vi "MainVI.vi"() -> ()   [LabVIEW 2020]
uses:
  System.Speech
panel:
  in  "WITHDRAW":bool
  in  "PIN ENTER":bool
  in  "Keyboard":T1
  in  "NAME ENTER":bool
  in  "RUN":bool
  in  "INSERT CARD":bool
  out "Screen":string
  # "PROJECT"
  # "VIRTUAL ATM"
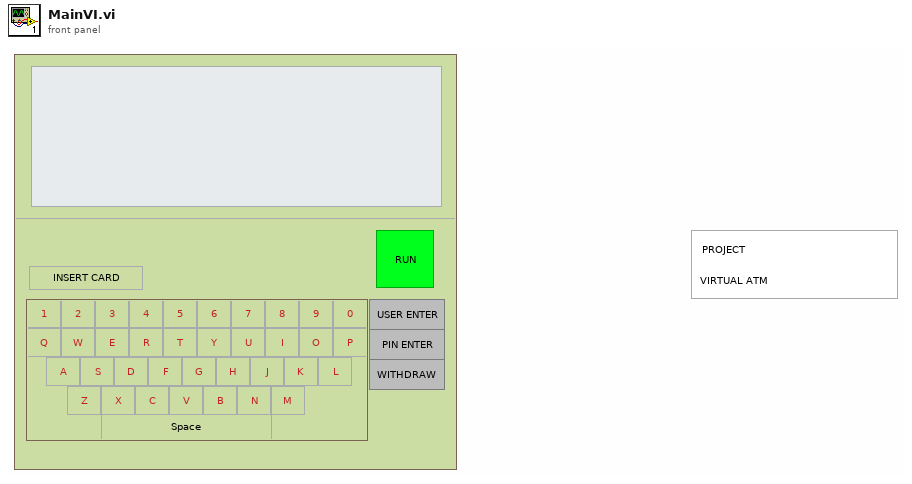
[diagram p1: front panel]
types:
  T1 = cluster{"Q":bool, "W":bool, "E":bool, "R":bool, "T":bool, "Y":bool, "U":bool, "I":bool, "O":bool, "P":bool, "A":bool, "S":bool, "D":bool, "F":bool, "G":bool, "H":bool, "J":bool, "K":bool, "L":bool, "Z":bool, "X":bool, "C":bool, "V":bool, "B":bool, "N":bool, "M":bool, "1":bool, "2":bool, "3":bool, "4":bool, "5":bool, "6":bool, "7":bool, "8":bool, "9":bool, "0":bool, bool}
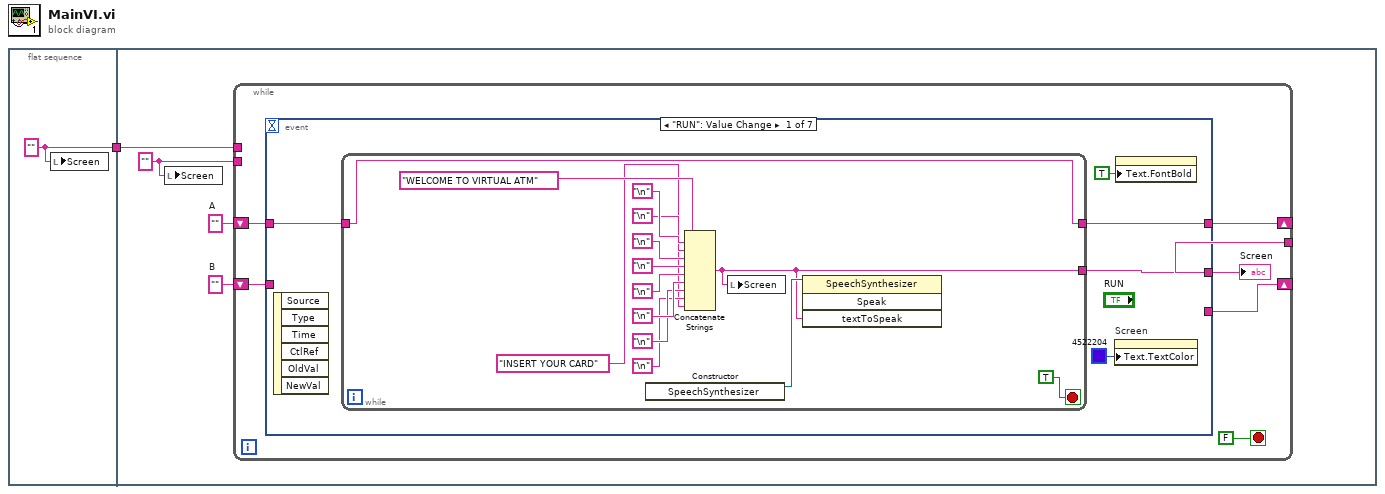
[diagram p0: block diagram]
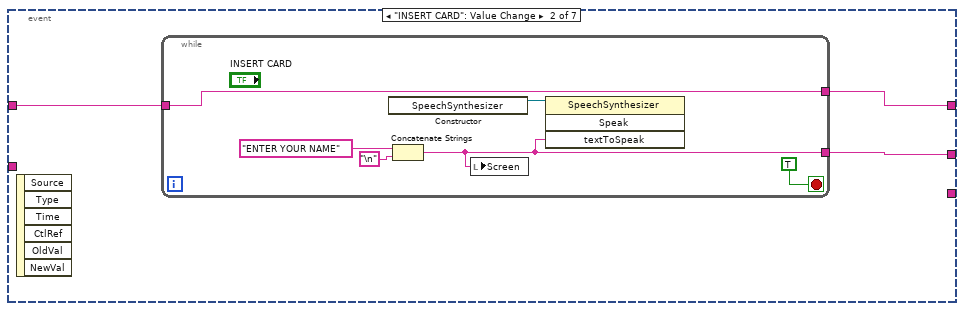
[diagram p2: hidden frame]
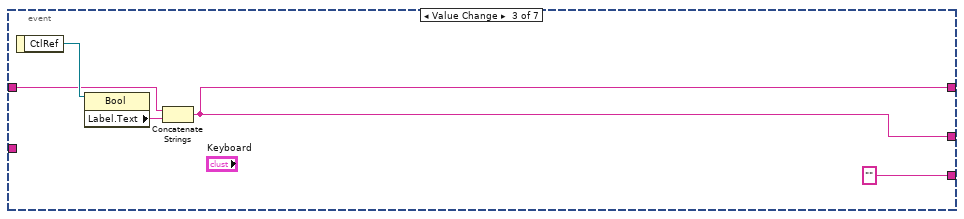
[diagram p3: hidden frame]
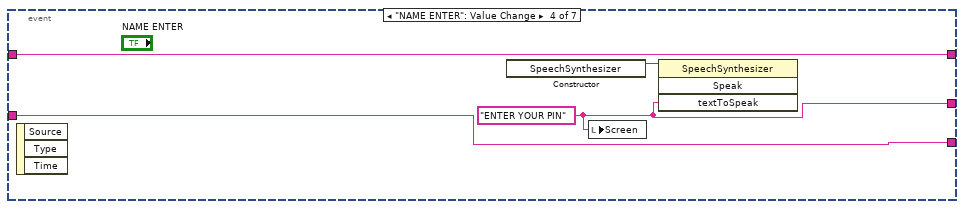
[diagram p4: hidden frame]
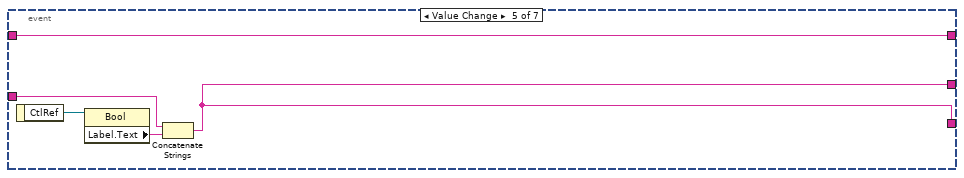
[diagram p5: hidden frame]
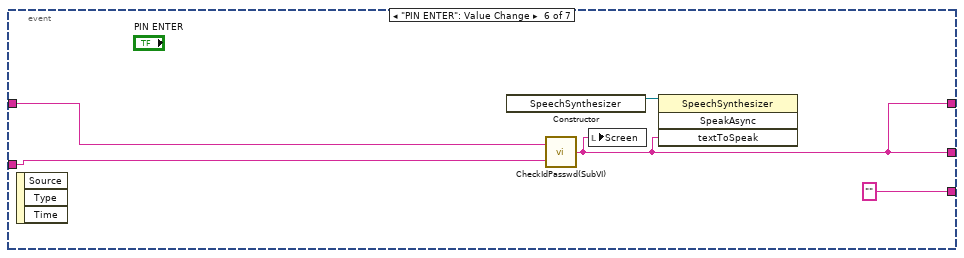
[diagram p6: hidden frame]
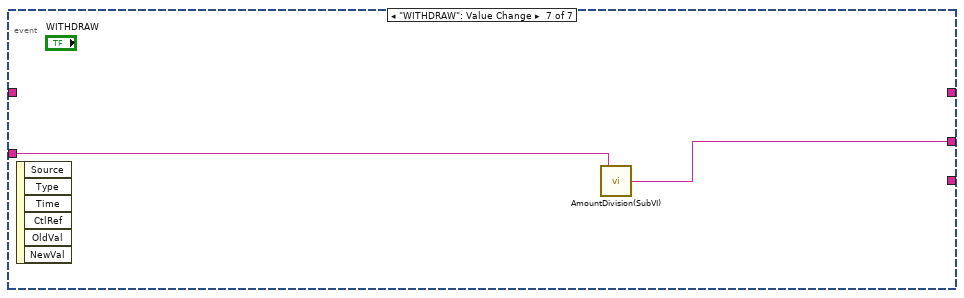
[diagram p7: hidden frame]
diagram:
  n1 = flat-sequence {
    tunnel: [w2] -> w1
    tunnel: w1 -> [w6]
    frame #0 {
      w2 = "" ("Screen")
      n2 = local write "Screen"(w2) -> ()
    }
    frame #1 {
      w3 = ""
      w4 = ""  # A
      w5 = ""  # B
      n3 = local write "Screen"(w3) -> ()
      n4 = while {
        shift-right: [w12] -> _
        shift-left: w5 -> [w11]
        tunnel: w6 -> [_]
        shift-right: [w10] -> _
        shift-left: w4 -> [w8]
        tunnel: w3 -> [_]
        tunnel: [w9] -> _
        stop <- FALSE stop-if-true
        n5 = event shown="[0] \"RUN\": Value Change" {
          selector: _ -> [_ _ _ _ _ _ _]
          dyn-events: _ -> [_ _ _ _ _ _ _]
          timeout: _ -> [_ _ _ _ _ _ _]
          tunnel: w11 -> [_ _ _ w46 w50 w59 w61]
          tunnel: [_ _ "" ("B") w46 w53 "" ("B") _] -> w12
          tunnel: [w17 w34 w41 w48 w53 w55 w60] -> w9
          tunnel: w8 -> [w16 w33 w42 w47 w51 w58 _]
          tunnel: [w15 w32 w41 w47 w51 w55 _] -> w10
          event "RUN": Value Change {
            n6 = event-data() -> ()  [unwired: 1 in, 6 out]
            n7 = while {
              tunnel: [w19] -> w17
              tunnel: w16 -> [w18]
              tunnel: [w18] -> w15
              stop <- TRUE stop-if-true
              n8 = constructor class="SpeechSynthesizer"() -> (reference out=w31:refnum<k24>)  [unwired: 3 in, 2 out]
              n9 = Concatenate Strings("WELCOME TO VIRTUAL ATM", "\n", "\n", "\n", "\n", "\n", "\n", "\n", "\n", "INSERT YOUR CARD" ("Screen")) -> (w19:string)
              n10 = local write "Screen"(w19) -> ()
              n11 = invoke class="SpeechSynthesizer" method="Speak"(reference=w31, "textToSpeak"=w19) -> ()  [unwired: 2 in, 4 out]
            }
            n12 = property on="Screen" class="Str"("Text.TextColor"=u32 4522204 ("Text.Text Colors:Text Color")) -> ()  [unwired: 2 in, 2 out]
            n13 = property on="Screen" class="Str"("Text.FontBold"=TRUE ("Text.Font:Bold")) -> ()  [unwired: 2 in, 2 out]
          }
          event "INSERT CARD": Value Change {
            n14 = event-data() -> ()  [unwired: 1 in, 6 out]
            n15 = while {
              tunnel: [w37] -> w34
              tunnel: [w35] -> w32
              tunnel: w33 -> [w35]
              stop <- TRUE stop-if-true
              n16 = constructor class="SpeechSynthesizer"() -> (reference out=w40:refnum<k24>)  [unwired: 3 in, 2 out]
              n17 = Concatenate Strings("ENTER YOUR NAME" ("string"), "\n") -> (w37:string)
              n18 = local write "Screen"(w37) -> ()
              n19 = invoke class="SpeechSynthesizer" method="Speak"(reference=w40, "textToSpeak"=w37) -> ()  [unwired: 2 in, 4 out]
            }
          }
          event "Keyboard.", "Keyboard.W", "Keyboard.E", "Keyboard.R", "Keyboard.T", "Keyboard.Y", "Keyboard.U", "Keyboard.I", "Keyboard.O", "Keyboard.P", "Keyboard.A", "Keyboard.S", "Keyboard.D", "Keyboard.F", "Keyboard.G", "Keyboard.H", "Keyboard.J", "Keyboard.K", "Keyboard.L", "Keyboard.Z", "Keyboard.X", "Keyboard.C", "Keyboard.V", "Keyboard.B", "Keyboard.N": Value Change {
            n20 = event-data() -> ("CtlRef"=w44:refnum<vi>)  [unwired: 1 in]
            n21 = property class="Bool"(reference=w44) -> ("Label.Text"=w45:string)  [unwired: 1 in, 2 out]
            n22 = Concatenate Strings(w42, w45) -> (w41:string)
          }
          event "NAME ENTER": Value Change {
            w48 = "ENTER YOUR PIN"
            n23 = event-data() -> ()  [unwired: 1 in, 3 out]
            n24 = constructor class="SpeechSynthesizer"() -> (reference out=w49:refnum<k24>)  [unwired: 3 in, 2 out]
            n25 = local write "Screen"(w48) -> ()
            n26 = invoke class="SpeechSynthesizer" method="Speak"(reference=w49, "textToSpeak"=w48) -> ()  [unwired: 2 in, 4 out]
          }
          event "Keyboard.1", "Keyboard.2", "Keyboard.3", "Keyboard.4", "Keyboard.5", "Keyboard.6", "Keyboard.7", "Keyboard.8", "Keyboard.9", "Keyboard.0": Value Change {
            n27 = event-data() -> ("CtlRef"=w54:refnum<vi>)  [unwired: 1 in]
            n28 = property class="Bool"(reference=w54) -> ("Label.Text"=w52:string)  [unwired: 1 in, 2 out]
            n29 = Concatenate Strings(w50, w52) -> (w53:string)
          }
          event "PIN ENTER": Value Change {
            n30 = event-data() -> ()  [unwired: 1 in, 3 out]
            n31 = constructor class="SpeechSynthesizer"() -> (reference out=w56:refnum<k24>)  [unwired: 3 in, 2 out]
            n32 = call "CheckIdPasswd(SubVI).vi"("PIN"=w59, "User Name"=w58) -> ("output"=w55:string)
            n33 = local write "Screen"(w55) -> ()
            n34 = invoke class="SpeechSynthesizer" method="SpeakAsync"(reference=w56, "textToSpeak"=w55) -> ()  [unwired: 2 in, 4 out]
          }
          event "WITHDRAW": Value Change {
            n35 = event-data() -> ()  [unwired: 1 in, 6 out]
            n36 = call "AmountDivision(SubVI).vi"("Amount"=w61) -> ("output"=w60:string)
          }
        }
        "Screen" <- w9
      }
    }
  }
